vi "subVI_pulseArray.vi"(11 "Brightness":u8) -> (3 "Pulsearray":i32[](array[numeric]))   [LabVIEW 2018, in "HASS-LV-WS_integration.lvlib"]
uses:
  HASS-LV-WS_integration.lvlib
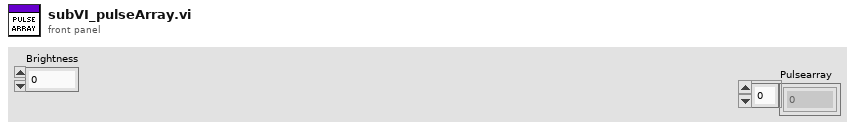
[diagram p1: front panel]
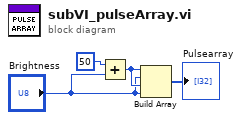
[diagram p0: block diagram]
diagram:
  n1 = Add(x=u8 50, y="Brightness") -> (x+y=w2:u8)
  n2 = Build Array(w2, "Brightness", w2, "Brightness") -> (→"Pulsearray":u8[])
